vi "Get New Range.vi"(0 "Ranges":string[](array[string]), 1 "Range (numeric)":dbl[](array[numeric]), 2 "Range (char)":string, 3 "Action":i32(ring) items=["Decrease"=-1, "Increase"=1, "None"=0]) -> (7 "New Range":string, 9 "New?":bool)   [LabVIEW 2009]
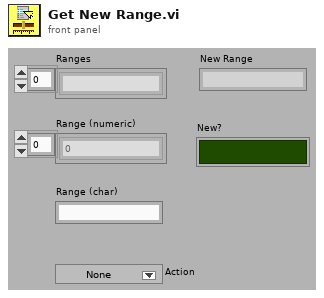
[diagram p1: front panel]
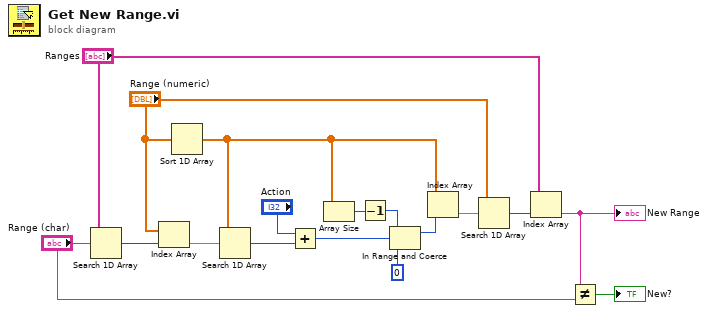
[diagram p0: block diagram]
diagram:
  n1 = Search 1D Array(1D array="Ranges", element="Range (char)") -> (index of element=w10:i32)  [unwired: 1 in]
  n2 = Index Array(array="Range (numeric)", index=w10) -> (element=w9:dbl)
  n3 = Sort 1D Array(array="Range (numeric)") -> (sorted array=w13:dbl[])
  n4 = Search 1D Array(1D array=w13, element=w9) -> (index of element=w3:i32)  [unwired: 1 in]
  n5 = Add(x="Action", y=w3) -> (x+y=w1:i32)
  n6 = Array Size(array=w13) -> (size(s)=w17:i32)
  n7 = Decrement(x=w17) -> (x-1=w16:i32)
  n8 = In Range and Coerce(upper limit=w16, x=w1, lower limit=0) -> (coerced(x)=w14:i32)  [unwired: 1 out]
  n9 = Index Array(array=w13, index=w14) -> (element=w12:dbl)
  n10 = Search 1D Array(1D array="Range (numeric)", element=w12) -> (index of element=w11:i32)  [unwired: 1 in]
  n11 = Index Array(array="Ranges", index=w11) -> (element=w5:string)
  "New Range" <- w5
  n12 = Not Equal?(x=w5, y="Range (char)") -> (x != y?=→"New?":bool)
